vi "tm_getarea_a.vi"(8 "error in (no error)":errorcluster, 11 "Handle in":u32) -> (0 "error out":errorcluster, 1 "V Offset":T1, 2 "H Offset":T1, 3 "Handle out":u32, 4 "H Width":T1, 6 "V Width":T1)   [LabVIEW 2015]
uses:
  tmcamcon.dll
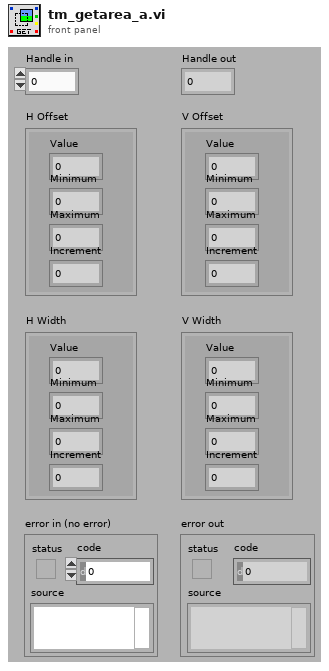
[diagram p1: front panel]
types:
  T1 = cluster{"Value":i32, "Minimum":i32, "Maximum":i32, "Increment":i32}
  T2 = cluster{"hov":i32, "hon":i32, "hox":i32, "hoi":i32}
  T3 = cluster{"hwv":i32, "hwn":i32, "hwx":i32, "hwi":i32}
  T4 = cluster{"vov":i32, "von":i32, "vox":i32, "voi":i32}
  T5 = cluster{"vwv":i32, "vwn":i32, "vwx":i32, "vwi":i32}
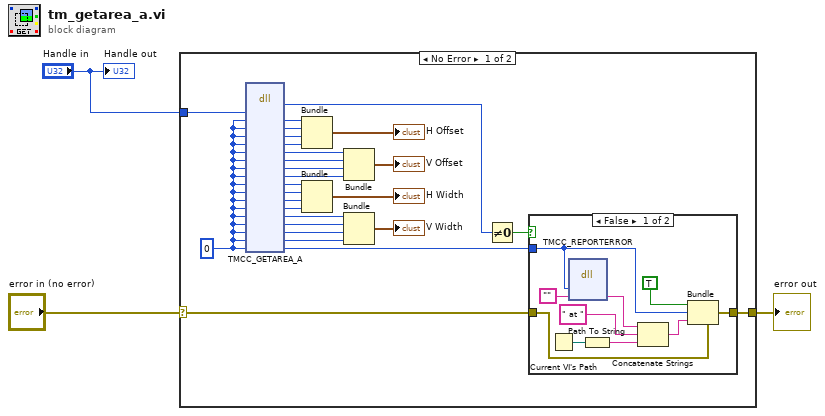
[diagram p0: block diagram]
diagram:
  n1 = case shown="No Error" "error in (no error)" {
    selector: "error in (no error)" -> [w22 w42]
    tunnel: [w21 w42] -> w2
    tunnel: "Handle in" -> [w4 _]
    frame No Error {
      w20 = 0
      n2 = dll-call lib="tmcamcon.dll" fn="TMCC_GETAREA_A"("index"=w4, "hov"=w20, "hon"=w20, "hox"=w20, "hoi"=w20, "vov"=w20, "von"=w20, "vox"=w20, "voi"=w20, "hwv"=w20, "hwn"=w20, "hwx"=w20, "hwi"=w20, "vwv"=w20, "vwn"=w20, "vwx"=w20, "vwi"=w20, "Erval"=w20) -> ("return type"=w30:u32, "hov"=w27:i32, "hon"=w28:i32, "hox"=w29:i32, "hoi"=w26:i32, "vov"=w19:i32, "von"=w18:i32, "vox"=w17:i32, "voi"=w16:i32, "hwv"=w15:i32, "hwn"=w14:i32, "hwx"=w13:i32, "hwi"=w12:i32, "vwv"=w11:i32, "vwn"=w10:i32, "vwx"=w9:i32, "vwi"=w8:i32, "Erval"=w23:i32)  [unwired: 4 in, 2 out]
      n3 = Bundle("hov"=w27, "hon"=w28, "hox"=w29, "hoi"=w26) -> (→"H Offset":T2)  [unwired: 1 in]
      n4 = Bundle("hwv"=w15, "hwn"=w14, "hwx"=w13, "hwi"=w12) -> (→"H Width":T3)  [unwired: 1 in]
      n5 = Bundle("vov"=w19, "von"=w18, "vox"=w17, "voi"=w16) -> (→"V Offset":T4)  [unwired: 1 in]
      n6 = Bundle("vwv"=w11, "vwn"=w10, "vwx"=w9, "vwi"=w8) -> (→"V Width":T5)  [unwired: 1 in]
      n7 = Not Equal To 0?(x=w30) -> (x != 0?=w24:bool)
      n8 = case shown="False" w24 {
        tunnel: w22 -> [w40 w41]
        tunnel: [w39 w41] -> w21
        tunnel: w23 -> [w33 _]
        frame False {
          n9 = Current VI's Path() -> (path=w38:path)
          n10 = dll-call lib="tmcamcon.dll" fn="TMCC_REPORTERROR"("error"=w33, "buf"="") -> ("buf"=w32:string)  [unwired: 5 in, 2 out]
          n11 = Path To String(path=w38) -> (string=w34:string)
          n12 = Concatenate Strings(w32, " at ", w34) -> (w37:string)
          n13 = Bundle(cluster=w40, "status"=TRUE, "code"=w33, "source"=w37) -> (w39:errorcluster)
        }
        frame True {
        }
      }
    }
    frame Error {
    }
  }
  "error out" <- w2
  "Handle out" <- "Handle in"
